vi "Tektronix TDS 3000 Series Single Channel Waveform Acquire.vi"() -> ()   [LabVIEW 2010]
doc: "DESCRIPTION:\nThis VI shows how to configure the Tektronix TDS 3xxx Series for a single-channel waveform acquisition. It uses edge triggering to trigger the acquisition. \n\nINSTRUCTIONS:\n1. Pass a valid VISA session\n2. Enter a vertical offset, range and coupling for the specified channel.\n3. Enter the probe attenuation for the probe attached to the specified channel input.\n4. Enter the acquisition start time and desired time per record.\n5. Enter the trigger level for the edge trigger.\n6. Run the VI.\n7. The acquired waveform will be displayed in the graph.\n\nNOTES:\nNotice the order of the Tektronix tktds3k component VIs in the block diagram.\n\nThis VI sets the following controls on the block diagram:\n 20MHz Max Input Frequency.\n 1.0M Ohm Input Impedance.\n 500ns trigger holdoff.\n Edge trigger is DC coupled with a positive slope.\nTo change these controls, modify the associated block diagram constants."
uses:
  <instrlib>/Tektronix TDS 3000 Series/Tektronix TDS 3000 Series.lvlib
panel:
  in  "Trigger Source (Chan 1)":string(combo)="CH1"
  in  "Trigger Level  (1.0 V)":dbl=1.0 format="%.2p"
  in  "Time Per Record (4.0E-3 s)":dbl=0.004 format="%.2p"
  in  "Acquisition Start Time (0.0 s)":dbl format="%.2p"
  in  "Vertical Coupling (DC)":i32(slide)=1
  in  "Probe Attenuation (1.0)":dbl=1.0 format="%.2f"
  in  "Channel (\"CH1\")":string(combo)="CH1"
  in  "Vertical Range (10.0 V)":dbl=10.0 format="%.2p"
  in  "Vertical Offset (0.0 V)":dbl format="%.3p"
  in  "VISA resource name":refnum<visa-resource-name>="GPIB0::1::INSTR"
  out "Waveform Graph":T1(graph)
  # "© 2003-2006, National Instruments, Corporation.  All Rights Reserved."
  # "For instructions,\nselect Show Context Help\nfrom the Help menu."
  # "Channel Configuration"
  # "Horizontal Configuration"
  # "Triggering"
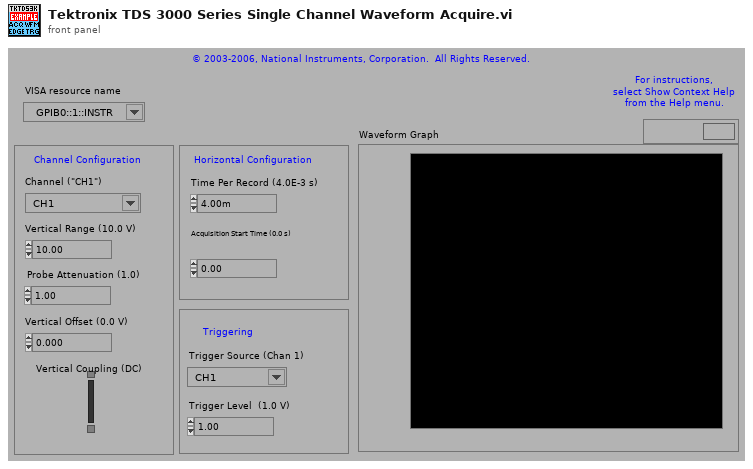
[diagram p1: front panel]
types:
  T1 = cluster{"Initial X":dbl, "X Increment":dbl, "Waveform Array":dbl[]}
  T2 = cluster{"Baud Rate (9600)":u32, "Flow Control (RTS/CTS)":u16, i32}
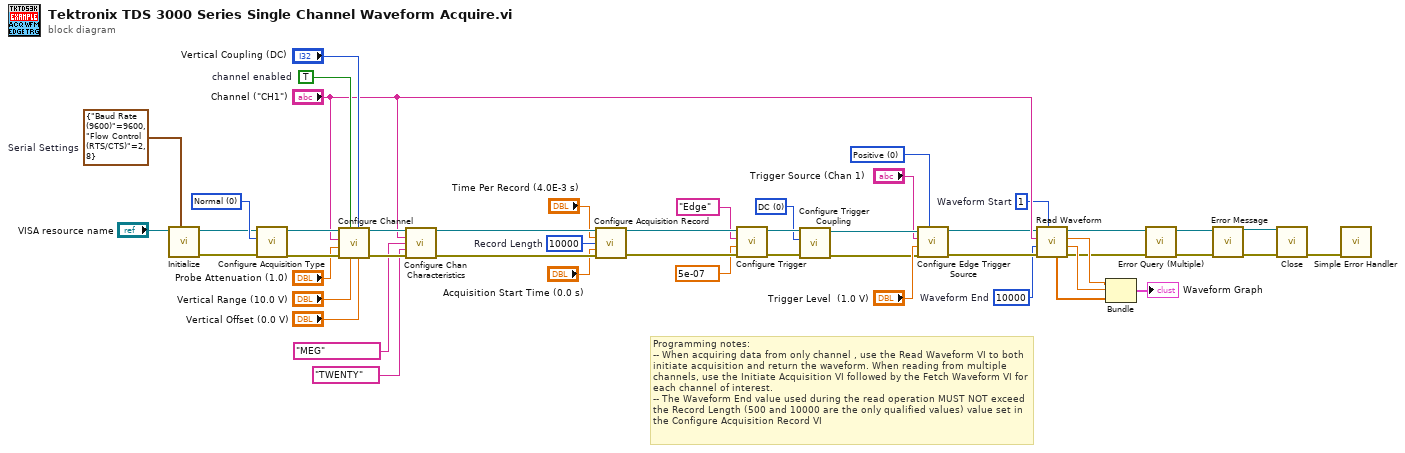
[diagram p0: block diagram]
diagram:
  w2 = 1  # Waveform Start
  w3 = 10000  # Waveform End
  w4 = 10000  # Record Length
  w15 = T2 {"Baud Rate (9600)"=9600, "Flow Control (RTS/CTS)"=2, 8}  # Serial Settings
  w24 = 0 items=["Normal", "Peak Detect", "Envelope", "Average"] ("Acquisition Type (0:Normal)")
  w27 = u32 0 items=["DC", "High Frequency Reject", "Low Frequency Reject", "Noise Reject"] ("Trigger Coupling (DC)")
  w28 = 0 items=["Positive", "Negative"] ("Trigger Slope (Positive)")
  w35 = TRUE  # channel enabled
  # "Programming notes:\n-- When acquiring data from only channel , use the Read Waveform VI to both initiate acquisition and return the waveform. When reading from multiple channels, use the Initiate Acquisition VI followed by the Fetch Waveform VI for each channel of interest. \n-- The Waveform End value used during the read operation MUST NOT exceed the Record Length (500 and 10000 are the only qualified values) value set in the Configure Acquisition Record VI"
  n1 = call <instrlib>:"Initialize.vi"("Serial Settings"=w15, "VISA Resource Name"="VISA resource name") -> ("error out"=w17:errorcluster, "VISA Resource Name Out"=w18:refnum<visa-resource-name>)  [unwired: 8 in]
  n2 = call <instrlib>:"Configure Acquisition Type.vi"("error in (no error)"=w17, "Acquisition Type (0:Sample)"=w24, "VISA Resource Name"=w18) -> ("error out"=w49:errorcluster, "VISA Resource Name Out"=w47:refnum<visa-resource-name>)  [unwired: 7 in]
  n3 = call <instrlib>:"Configure Channel.vi"("Vertical Offset (0.0 V)"="Vertical Offset (0.0 V)", "Vertical Coupling (DC)"="Vertical Coupling (DC)", "Vertical Range (10.0 V)"="Vertical Range (10.0 V)", "Channel Enabled (True)"=w35, "error in (no error)"=w49, "Probe Attenuation (1.0)"="Probe Attenuation (1.0)", "Channel Name (\"CH1\")"="Channel (\"CH1\")", "VISA Resource Name"=w47) -> ("error out"=w48:errorcluster, "VISA Resource Name Out"=w46:refnum<visa-resource-name>)  [unwired: 2 in]
  n4 = call <instrlib>:"Configure Chan Characteristics.vi"("VISA Resource Name"=w46, "Channel Name (\"CH1\")"="Channel (\"CH1\")", "Input Impedance (1.0 mega ohm)"="MEG", "Max Input Frequency (20.0E+6 Hz)"="TWENTY", "error in (no error)"=w48) -> ("VISA Resource Name Out"=w43:refnum<visa-resource-name>, "error out"=w42:errorcluster)  [unwired: 9 in]
  n5 = call <instrlib>:"Configure Acquisition Record.vi"("VISA Resource Name"=w43, "Time Per Record (4.0e-3 s)"="Time Per Record (4.0E-3 s)", "Record Length (10000)"=w4, "Acquisition Start Time (0.0 s)"="Acquisition Start Time (0.0 s)", "error in (no error)"=w42) -> ("VISA Resource Name Out"=w41:refnum<visa-resource-name>, "error out"=w40:errorcluster)  [unwired: 9 in]
  n6 = call <instrlib>:"Configure Trigger.vi"("error in (no error)"=w40, "Trigger Holdoff (0.00 sec)"=5e-07 ("trigger holdoff (500ns)"), "Trigger Type (Edge)"="Edge", "VISA Resource Name"=w41) -> ("error out"=w30:errorcluster, "VISA Resource Name Out"=w32:refnum<visa-resource-name>)  [unwired: 6 in]
  n7 = call <instrlib>:"Configure Trigger Coupling.vi"("error in (no error)"=w30, "Trigger Coupling (DC)"=w27, "VISA Resource Name"=w32) -> ("error out"=w29:errorcluster, "VISA Resource Name Out"=w31:refnum<visa-resource-name>)  [unwired: 7 in]
  n8 = call <instrlib>:"Configure Edge Trigger Source.vi"("Trigger Slope (Positive)"=w28, "error in (no error)"=w29, "Trigger Level (0.0 V)"="Trigger Level  (1.0 V)", "Trigger Source (Channel 1)"="Trigger Source (Chan 1)", "VISA Resource Name"=w31) -> ("error out"=w6:errorcluster, "VISA Resource Name Out"=w7:refnum<visa-resource-name>)  [unwired: 5 in]
  n9 = call <instrlib>:"Read Waveform.vi"("Waveform Start (1)"=w2, "error in (no error)"=w6, "Waveform End (10000)"=w3, "Source (Channel 1)"="Channel (\"CH1\")", "VISA Resource Name"=w7) -> ("error out"=w13:errorcluster, "X Increment"=w21:dbl, "Initial X"=w20:dbl, "VISA Resource Name Out"=w14:refnum<visa-resource-name>, "Waveform Array"=w22:dbl[])  [unwired: 1 in, 1 out]
  n10 = Bundle("Initial X"=w20, "X Increment"=w21, "Waveform Array"=w22) -> (→"Waveform Graph":T1)  [unwired: 1 in]
  n11 = call <instrlib>:"Error Query (Multiple).vi"("error in (no error)"=w13, "VISA Resource Name"=w14) -> ("error out"=w11:errorcluster, "VISA Resource Name Out"=w12:refnum<visa-resource-name>)  [unwired: 6 in, 2 out]
  n12 = call <instrlib>:"Error Message.vi"("VISA Resource Name"=w12, "error in (no error)"=w11) -> ("VISA Resource Name Out"=w10:refnum<visa-resource-name>, "error out"=w9:errorcluster)  [unwired: 9 in, 3 out]
  n13 = call <instrlib>:"Close.vi"("error in (no error)"=w9, "VISA Resource Name"=w10) -> ("error out"=w8:errorcluster)  [unwired: 9 in]
  n14 = call <vilib>:"Simple Error Handler.vi"("error in (no error)"=w8) -> ()  [unwired: 4 in, 5 out]
